vi "Get DefaultValue.vi"(11 "Object Type in":refnum<class "Object Type Base.lvclass">) -> (1 "Defined?":bool, 2 "DefaultValue":string, 3 "Object Type out":refnum<class "Object Type Base.lvclass">)   [LabVIEW 2024, in "EDS.lvlib" / "Object Type Base.lvclass"]
uses:
  Object Type Base.lvclass
  Object Type Base.lvclass/Object Type Base.ctl
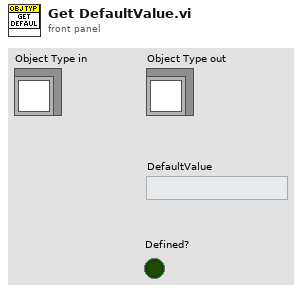
[diagram p1: front panel]
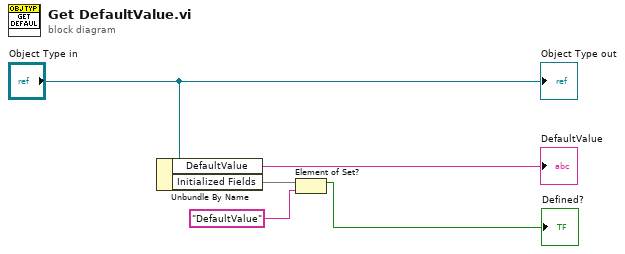
[diagram p0: block diagram]
diagram:
  n1 = Unbundle By Name("Object Type in") -> ("DefaultValue"=→"DefaultValue":string, "Initialized Fields"=w3:set{string})
  n2 = Element of Set?(10:"DefaultValue" ("element"), 11:w3) -> (3:→"Defined?":bool)
  "Object Type out" <- "Object Type in"
